vi "AlazarFFTBackgroundSubtractionSetEnabled.vi"(3 "error in (no error)":errorcluster, 4 "Enabled":u32 format="%.0g", 5 "DSP Handle":u64) -> (0 "error out":errorcluster, 1 "Return Code":u32, 2 "DSP Handle":u64)   [LabVIEW 2018]
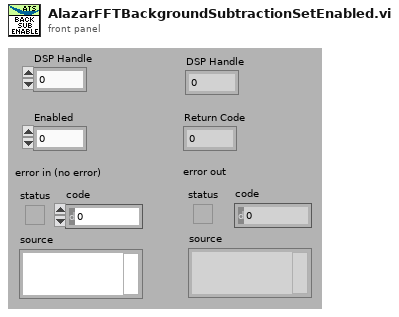
[diagram p1: front panel]
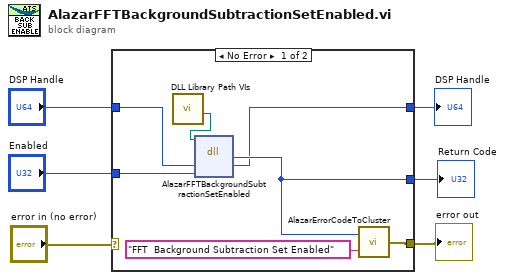
[diagram p0: block diagram]
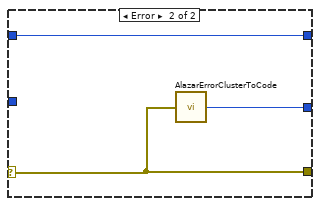
[diagram p2: hidden frame]
diagram:
  n1 = case shown="No Error" "error in (no error)" {
    selector: "error in (no error)" -> [_ w15]
    tunnel: [w11 w15] -> w4
    tunnel: [w13 w16] -> w3
    tunnel: [w10 w14] -> w5
    tunnel: "Enabled" -> [w9 _]
    tunnel: "DSP Handle" -> [w8 w14]
    frame No Error {
      n2 = call "DLL Library Path VIs.vi"() -> ("Alazar"=w7:path)  [unwired: 9 in, 2 out]
      n3 = dll-call lib="C:/Project/SerialSectOCT - FFT GPU/SerialSectOCT/Labview Software/DLL/ATSApi.dll" fn="AlazarFFTBackgroundSubtractionSetEnabled"(path in=w7, "dspHandle"=w8, "enabled"=w9) -> ("return type"=w13:u32, "dspHandle"=w10:u64)  [unwired: 3 in, 2 out]
      n4 = call "AlazarErrorCodeToCluster.vi"("Message"="FFT  Background Subtraction Set Enabled", "Error Code"=w13) -> ("error out"=w11:errorcluster)
    }
    frame Error {
      n5 = call "AlazarErrorClusterToCode.vi"("error in (no error)"=w15) -> ("Error Code"=w16:u32)
    }
  }
  "DSP Handle" <- w5
  "error out" <- w4
  "Return Code" <- w3
